vi "Basic Generate LV Icon Template Layer.vi"(8 "error in (no error)":errorcluster) -> (0 "error out":errorcluster, 2 "Picture":picture, 3 "Icon.lvlclass out":refnum<class "Icon.lvclass">)   [LabVIEW 2020]
doc: "Basic example that shows how to set the Template Layer."
uses:
  <vilib>/LabVIEW Icon API/lv_icon/Classes/Icon/Icon.lvclass
  <vilib>/LabVIEW Icon API/API_User Layer Data.ctl
  <vilib>/Utility/miscctls.llb/LVPoint32TypeDef.ctl
  <vilib>/picture/picture.llb/imagedata.ctl
  <vilib>/LabVIEW Icon API/API_Text.ctl
  <vilib>/LabVIEW Icon API/lv_icon/Controls/Pathes.ctl
  <vilib>/LabVIEW Icon API/LabVIEW Icon API.lvlib
  <vilib>/LabVIEW Icon API/lv_icon/lv_icon.lvlib
panel:
  out "output cluster":T1
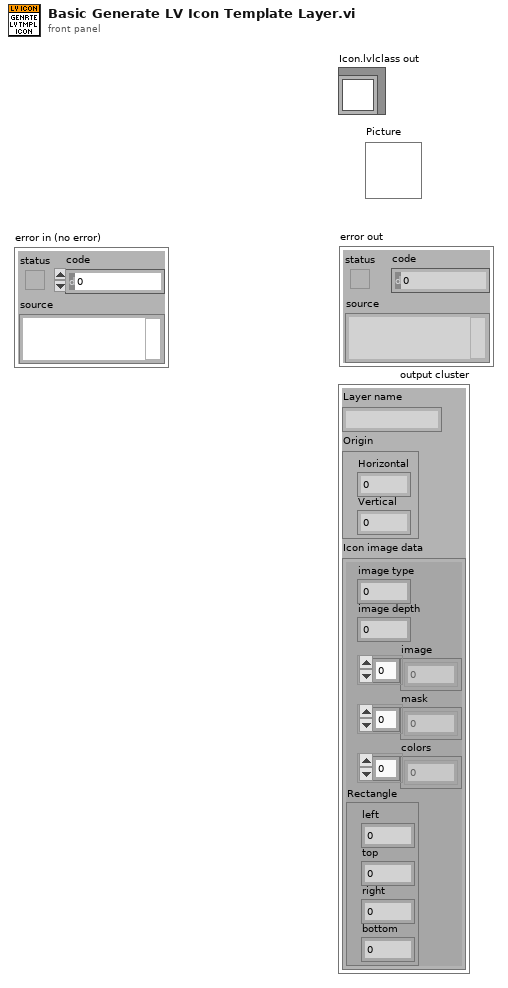
[diagram p1: front panel]
types:
  T1 = typedef "LabVIEW Icon API.lvlib/API_User Layer Data.ctl" = cluster{"Layer name":string, "Origin":T2, "Icon image data":T3}
  T2 = typedef "LVPoint32TypeDef.ctl" = cluster{"Horizontal":i32, "Vertical":i32}
  T3 = typedef "imagedata.ctl" = cluster{"image type":i32, "image depth":i32, "image":u8[], "mask":u8[], "colors":u32[], "Rectangle":cluster{"left":i16, "top":i16, "right":i16, "bottom":i16}}
  T4 = cluster{"left":i16, "top":i16, "right":i16, "bottom":i16}
  T5 = typedef "Pathes.ctl" = enum16{"Root Path", "Icon Templates", "Icon Templates VI", "Icon Templates Lib", "Glyphs"}
  T6 = typedef "LabVIEW Icon API.lvlib/API_Text.ctl" = cluster{"Line 1 text":string, "Line 2 text":string, "Line 3 text":string, "Line 4 text":string}
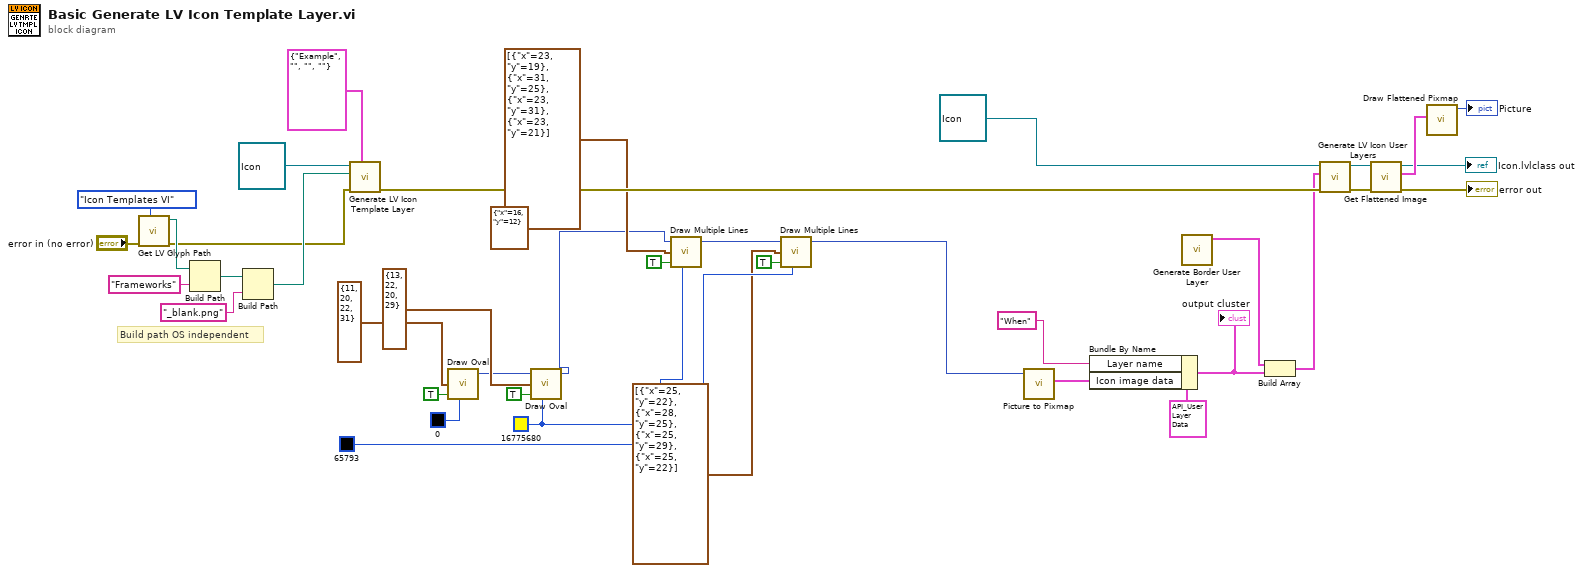
[diagram p0: block diagram]
diagram:
  w6 = u32 16775680 ("color(black)")
  (unwired) cluster{"x":i16, "y":i16} {"x"=16, "y"=12}
  # "Build path OS independent"
  n1 = call <vilib>:"Get LV Glyph Path.vi"("Path"=Pathes."Icon Templates VI", "error in (no error)"="error in (no error)") -> ("error out"=w20:errorcluster, "Requested Path"=w25:path)  [unwired: 1 in, 7 out]
  n2 = Build Path(base path=w25, name or relative path="Frameworks") -> (appended path=w23:path)
  n3 = Build Path(base path=w23, name or relative path="_blank.png") -> (appended path=w21:path)
  n4 = call <vilib>:"Generate LV Icon Template Layer.vi"("Text"=T6 {"Line 1 text"="Example", "Line 2 text"="", "Line 3 text"="", "Line 4 text"=""}, "error in (no error)"=w20, "Template path"=w21, "Icon.lvclass in"=refnum<class "Icon.lvclass"> refnum) -> ("error out"=w36:errorcluster)  [unwired: 6 in, 1 out]
  n5 = call <vilib>:"Draw Oval.vi"("rect"=T4 {"left"=11, "top"=20, "right"=22, "bottom"=31}, "fill?(F)"=TRUE, "color(black)"=u32 0) -> ("new picture"=w9:picture)  [unwired: 6 in]
  n6 = call <vilib>:"Draw Oval.vi"("picture"=w9, "rect"=T4 {"left"=13, "top"=22, "right"=20, "bottom"=29}, "fill?(F)"=TRUE, "color(black)"=w6) -> ("new picture"=w13:picture)  [unwired: 5 in]
  n7 = call <vilib>:"Draw Multiple Lines.vi"("picture"=w13, "line endpoints"=cluster{"x":i16, "y":i16}[] [{"x"=23, "y"=19}, {"x"=31, "y"=25}, {"x"=23, "y"=31}, {"x"=23, "y"=21}], "fill?(F)"=TRUE, "color(black)"=u32 65793) -> ("new picture"=w8:picture)  [unwired: 5 in]
  n8 = call <vilib>:"Draw Multiple Lines.vi"("picture"=w8, "line endpoints"=cluster{"x":i16, "y":i16}[] [{"x"=25, "y"=22}, {"x"=28, "y"=25}, {"x"=25, "y"=29}, {"x"=25, "y"=22}], "fill?(F)"=TRUE, "color(black)"=w6) -> ("new picture"=w7:picture)  [unwired: 5 in]
  n9 = call <vilib>:"Picture to Pixmap.vi"("picture"=w7) -> ("image data"=w32:T3)  [unwired: 9 in, 1 out]
  n10 = Bundle By Name(cluster=T1 {"Layer name"="", "Origin"={"Horizontal"=0, "Vertical"=0}, "Icon image data"={"image type"=0, "image depth"=0, "image"=[], "mask"=[], "colors"=[], "Rectangle"={"left"=0, "top"=0, "right"=0, "bottom"=0}}} ("User layer"), "Layer name"="When", "Icon image data"=w32) -> (w30:T1)
  "output cluster" <- w30
  n11 = call <vilib>:"Generate Border User Layer.vi"() -> ("User Layer data"=w1:T1)  [unwired: 11 in]
  n12 = Build Array(w1, w30) -> (w2:T1[])
  n13 = call <vilib>:"Generate LV Icon User Layers.vi"("error in (no error)"=w36, "User layers"=w2, "Icon in"=refnum<class "Icon.lvclass"> refnum) -> ("error out"=w35:errorcluster, "Icon out"=w31:refnum<class "Icon.lvclass">)  [unwired: 7 in]
  n14 = call <vilib>:"Get Flattened Image.vi"("error in (no error)"=w35, "lv_icon.lvlib:Icon.lvclass in"=w31) -> ("error out"=→"error out":errorcluster, "Color Image"=w37:T3, "lv_icon.lvlib:Icon.lvclass out"=→"Icon.lvlclass out":refnum<class "Icon.lvclass">)  [unwired: 6 in, 1 out]
  n15 = call <vilib>:"Draw Flattened Pixmap.vi"("image data"=w37) -> ("new picture"=→"Picture":picture)  [unwired: 8 in]
